vi "Hardware config bundler-Boolean.vi"(7 "Keys setup.Boolean":T17, 8 "error in (no error)":errorcluster, 9 "Section name":string, 10 "Hardware Configuration I/P":T1={"Dev. PC"=FALSE, "Swap XY on stage"=FALSE, "No of AOD"=0, "Computer MAC address"="", "Externalise Triggers"=FALSE, "Trigger HW config"={"Available Device List"=0, "Device Address"=""}, "DAQmx Chan"={"Pockels AO"="", "Hard shutter AO"="", "PMT AOs"="", "Galvo AOs"="", "Power meter AI"=""}, "XY stage available"=FALSE, "XY Stage"={"COM port"="", "Baudrate"=0, "Type"=""}, "Z stage available"=FALSE, "Z Stage config cluster"={"COM port"="COM7", "Baudrate"=0, "Type"=""}, "Encoder available"=FALSE, "Encoder"={"IP address"="224.0.1.103", "Port"=7000, "Wheel radius (cm)"=16.0, "Encoder Trigger"=""}, "VidRec available"=FALSE, "Cam VidRec"={"DO flag-Video record"="", "DO flag-Trial start"=""}, "Laser Power Control HW config"={"Laser Power Control"="", "Laser Power Modulation Control"=enum."NI"}, "Laser 1 available"=FALSE, "Laser 1 config cluster"={"COM port"="COM7", "Baud Rate"=0, "Type"=""}, "Prechirper 1 available"=FALSE, "Prechirper 1 config cluster"={"Type"="", "Baud Rate"=0, "COM port"="COM7"}, "Control system.FPGA available?"=FALSE, "Control Sys. HW config"={"Control system.FPGA Type"=enum."Virtex 5", "Control system.Network adapter name"="", "Control system.MAC address"="", "Control system.Ethernet Port"=0, "Control system.Ethernet Port Opened"=FALSE}, "DAQ FPGA HW Config"={"FGPA Ref"=refnum, "Target"="RIO0", "input card type"=enum."AC Card"}} {"Encoder"."Wheel radius (cm)" format="%#_13g"}, 11 "Refnum in":T16) -> (0 "error out":errorcluster, 2 "Hardware Configuration O/P":T1={"Dev. PC"=FALSE, "Swap XY on stage"=FALSE, "No of AOD"=0, "Computer MAC address"="", "Externalise Triggers"=FALSE, "Trigger HW config"={"Available Device List"=0, "Device Address"=""}, "DAQmx Chan"={"Pockels AO"="", "Hard shutter AO"="", "PMT AOs"="", "Galvo AOs"="", "Power meter AI"=""}, "XY stage available"=FALSE, "XY Stage"={"COM port"="", "Baudrate"=0, "Type"=""}, "Z stage available"=FALSE, "Z Stage config cluster"={"COM port"="COM7", "Baudrate"=0, "Type"=""}, "Encoder available"=FALSE, "Encoder"={"IP address"="224.0.1.103", "Port"=7000, "Wheel radius (cm)"=16.0, "Encoder Trigger"=""}, "VidRec available"=FALSE, "Cam VidRec"={"DO flag-Video record"="", "DO flag-Trial start"=""}, "Laser Power Control HW config"={"Laser Power Control"="", "Laser Power Modulation Control"=enum."NI"}, "Laser 1 available"=FALSE, "Laser 1 config cluster"={"COM port"="COM7", "Baud Rate"=0, "Type"=""}, "Prechirper 1 available"=FALSE, "Prechirper 1 config cluster"={"Type"="", "Baud Rate"=0, "COM port"="COM7"}, "Control system.FPGA available?"=FALSE, "Control Sys. HW config"={"Control system.FPGA Type"=enum."Virtex 5", "Control system.Network adapter name"="", "Control system.MAC address"="", "Control system.Ethernet Port"=0, "Control system.Ethernet Port Opened"=FALSE}, "DAQ FPGA HW Config"={"FGPA Ref"=refnum, "Target"="RIO0", "input card type"=enum."AC Card"}} {"Encoder"."Wheel radius (cm)" format="%#_13g"}, 3 "Refnum out":T16)   [LabVIEW 2017]
uses:
  Typedefs/Ini file interface (Boolean).ctl
  <vilib>/Utility/config.llb/Config Data RefNum.ctl
  Typedefs/Hardware Configuration settings.ctl
  Typedefs/Triggers HW config.ctl
  Typedefs/DAQmx physical channels cluster.ctl
  Typedefs/XY Stage config cluster.ctl
  Typedefs/Z Stage config cluster.ctl
  Typedefs/Encoder config cluster.ctl
  Typedefs/Cam VidRec HW config setup cluster.ctl
  Typedefs/Laser Power Control HW config.ctl
  Typedefs/Laser 1 config cluster.ctl
  Typedefs/PreChirper 1 config cluster.ctl
  Typedefs/Control Sys HW config cluster.ctl
  Typedefs/DAQ FPGA HW config cluster.ctl
  RIG-SPECIFIC FILES/FPGA Refs/FPGA Ref.ctl
  <vilib>/userdefined/High Color/nirio_resource_hc.ctl
  Typedefs/FPGA input type AC-DC.ctl
  <vilib>/Utility/config.llb/NI_LVConfig.lvlib
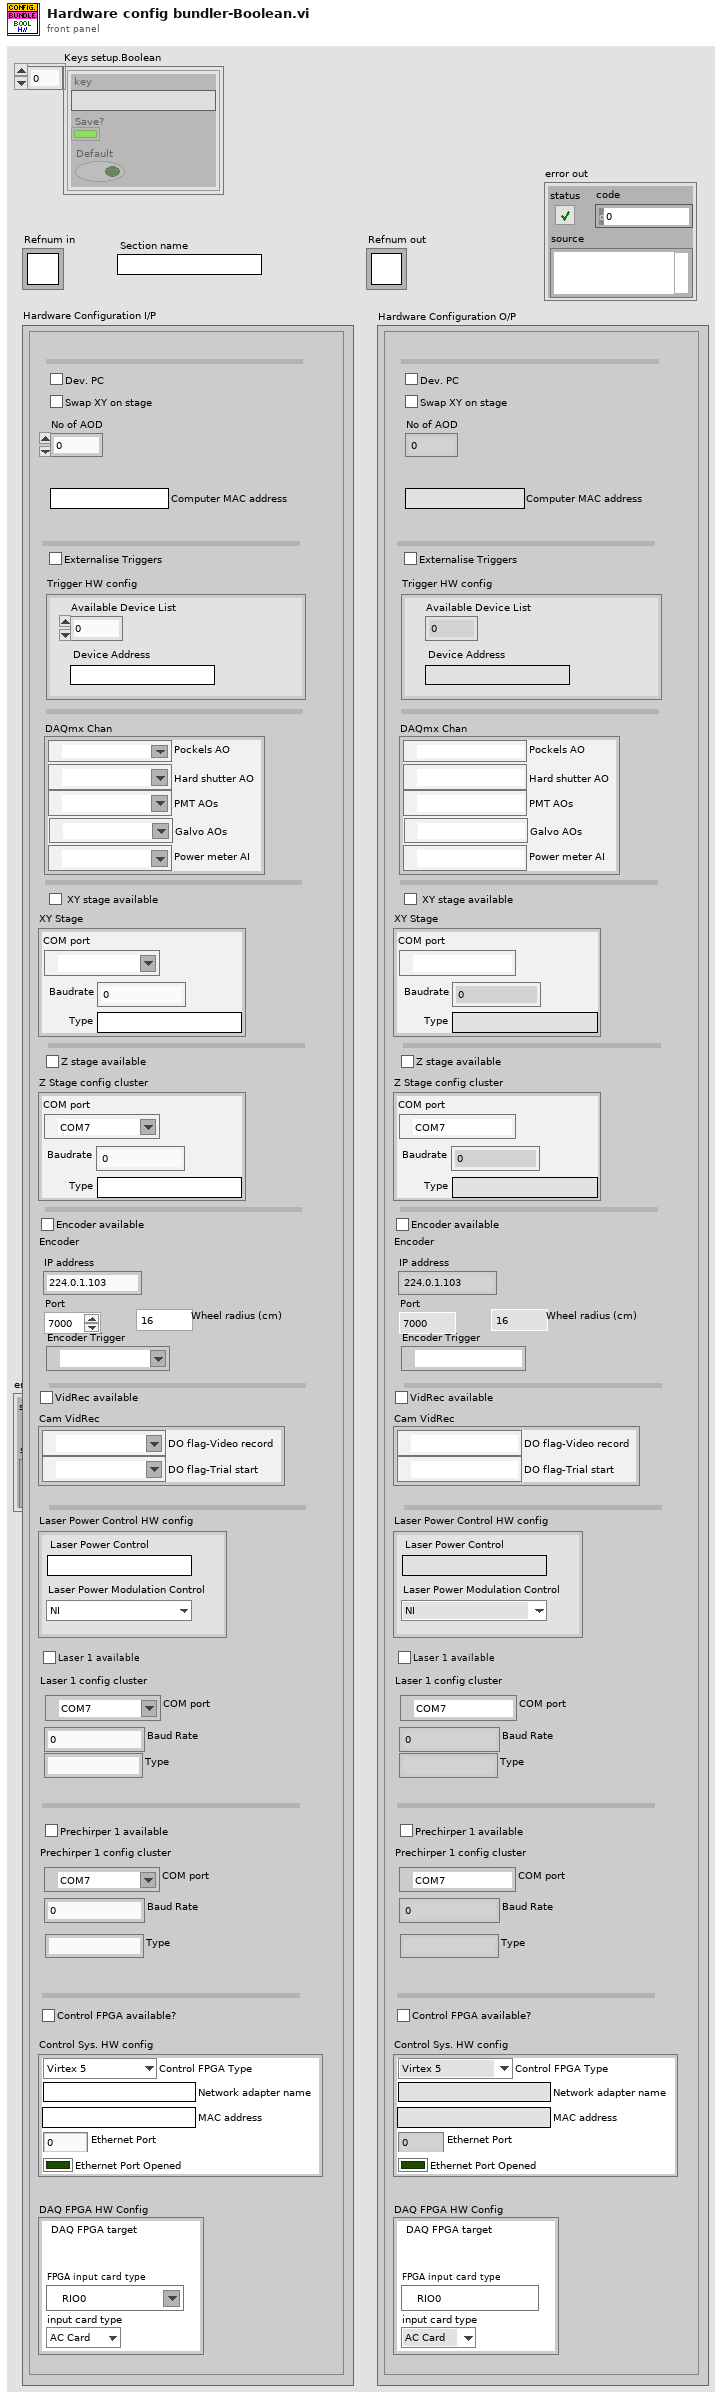
[diagram p1: front panel]
types:
  T1 = typedef "Hardware Configuration settings.ctl" = cluster{"Dev. PC":bool, "Swap XY on stage":bool, "No of AOD":u8, "Computer MAC address":string, "Externalise Triggers":bool, "Trigger HW config":T2, "DAQmx Chan":T3, "XY stage available":bool, "XY Stage":T4, "Z stage available":bool, "Z Stage config cluster":T5, "Encoder available":bool, "Encoder":T6, "VidRec available":bool, "Cam VidRec":T7, "Laser Power Control HW config":T8, "Laser 1 available":bool, "Laser 1 config cluster":T9, "Prechirper 1 available":bool, "Prechirper 1 config cluster":T10, "Control system.FPGA available?":bool, "Control Sys. HW config":T11, "DAQ FPGA HW Config":T12}
  T2 = typedef "Triggers HW config.ctl" = cluster{"Available Device List":i32, "Device Address":string}
  T3 = typedef "DAQmx physical channels cluster.ctl" = cluster{"Pockels AO":tag, "Hard shutter AO":tag, "PMT AOs":tag, "Galvo AOs":tag, "Power meter AI":tag}
  T4 = typedef "XY Stage config cluster.ctl" = cluster{"COM port":refnum<visa-resource-name>, "Baudrate":i32, "Type":string}
  T5 = typedef "Z Stage config cluster.ctl" = cluster{"COM port":refnum<visa-resource-name>, "Baudrate":i32, "Type":string}
  T6 = typedef "Encoder config cluster.ctl" = cluster{"IP address":string, "Port":u16, "Wheel radius (cm)":dbl, "Encoder Trigger":tag}
  T7 = typedef "Cam VidRec HW config setup cluster.ctl" = cluster{"DO flag-Video record":tag, "DO flag-Trial start":tag}
  T8 = typedef "Laser Power Control HW config.ctl" = cluster{"Laser Power Control":string, "Laser Power Modulation Control":enum16{"NI", "FPGA"}}
  T9 = typedef "Laser 1 config cluster.ctl" = cluster{"COM port":refnum<visa-resource-name>, "Baud Rate":i32, "Type":string}
  T10 = typedef "PreChirper 1 config cluster.ctl" = cluster{"Type":string, "Baud Rate":i32, "COM port":refnum<visa-resource-name>}
  T11 = typedef "Control Sys HW config cluster.ctl" = cluster{"Control system.FPGA Type":enum16{"Virtex 5", "Virtex 7"}, "Control system.Network adapter name":string, "Control system.MAC address":string, "Control system.Ethernet Port":u32, "Control system.Ethernet Port Opened":bool}
  T12 = typedef "DAQ FPGA HW config cluster.ctl" = cluster{"FGPA Ref":T13, "Target":T14, "input card type":T15}
  T13 = typedef "FPGA Ref.ctl" = refnum<k20>
  T14 = typedef "nirio_resource_hc.ctl" = tag
  T15 = typedef "FPGA input type AC-DC.ctl" = enum16{"AC Card", "DC Card"}
  T16 = typedef "NI_LVConfig.lvlib/Config Data RefNum.ctl" = refnum<k1>
  T17 = typedef "Ini file interface (Boolean).ctl" = cluster{"key":string, "Save?":bool, "Default":bool}[]
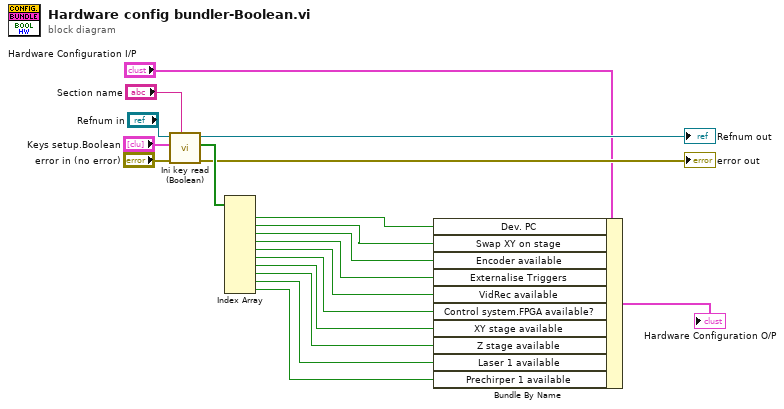
[diagram p0: block diagram]
diagram:
  n1 = call "Ini key read (Boolean).vi"("Section"="Section name", "error in (no error)"="error in (no error)", "Parameter names & setup"="Keys setup.Boolean", "Ini file refnum in"="Refnum in") -> ("error out"=→"error out":errorcluster, "Value read/used"=w18:bool[], "Ini file refnum out"=→"Refnum out":T16)  [unwired: 5 in]
  n2 = Index Array(array=w18) -> (element #1=w19:bool, element #2=w9:bool, element #3=w8:bool, element #4=w7:bool, element #5=w6:bool, element #6=w5:bool, element #7=w4:bool, element #8=w3:bool, element #9=w2:bool, element #10=w1:bool)  [unwired: 10 in]
  n3 = Bundle By Name(cluster="Hardware Configuration I/P", "Dev. PC"=w19, "Swap XY on stage"=w9, "Encoder available"=w8, "Externalise Triggers"=w7, "VidRec available"=w6, "Control system.FPGA available?"=w5, "XY stage available"=w4, "Z stage available"=w3, "Laser 1 available"=w2, "Prechirper 1 available"=w1) -> (→"Hardware Configuration O/P":T1)
